vi "Bld Cmd.vi"   [LabVIEW 2014, in "CN79000.lvclass"]
uses:
  CN79000.lvclass
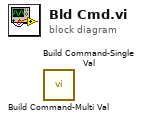
[diagram p0: block diagram]
diagram:
  n1 = call "Build Command-Multi Val.vi"() -> ()  [unwired: 7 in, 4 out]
  n2 = call "Build Command-Single Val.vi"() -> ()  [unwired: 7 in, 4 out]
